vi "Ophir_USBI_Test-2.00.vi"(2 "stop":bool) -> (14 "Power1 (W)":dbl format="%.3p")   [LabVIEW 2012]
panel:
  out "OphirPM":T1
  in  "Wait (mS)":u32=1000
  out "Power2 (W)":dbl(graph)=-5.33e-06
  out "error out":errorcluster
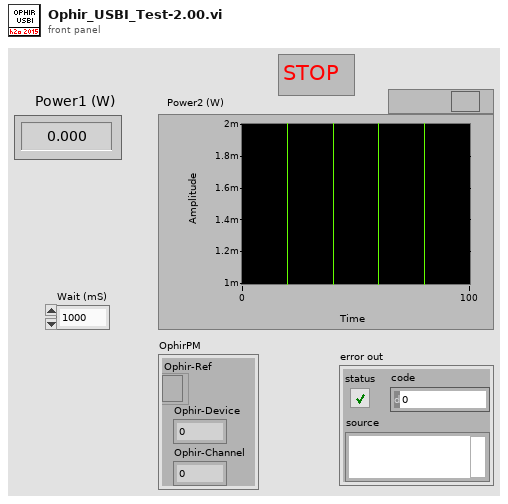
[diagram p1: front panel]
types:
  T1 = cluster{"Ophir-Ref":refnum<k7>, "Ophir-Device":i32, "Ophir-Channel":i32}
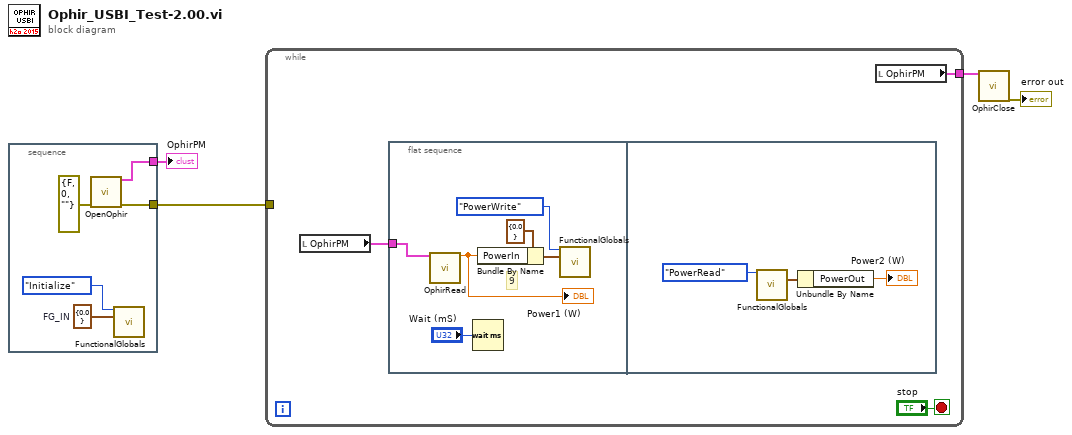
[diagram p0: block diagram]
diagram:
  n1 = stacked-sequence {
    tunnel: [w6] -> w1
    tunnel: [w5] -> w2
    frame #0 {
      w8 = cluster{"PowerIn":dbl} {"PowerIn"=0.0}  # FG_IN
      n2 = call "OpenOphir.vi"("error in (no error)"=errorcluster {"status"=FALSE, "code"=0, "source"=""}) -> ("OphirPM"=w6:T1, "error out"=w5:errorcluster)  [unwired: 13 in]
      n3 = call "FunctionalGlobals.vi"("FG_Control"=enum16{"Initialize", "PowerRead", "PowerWrite"}."Initialize", "FG_IN"=w8) -> ()  [unwired: 13 in, 1 out]
    }
  }
  "OphirPM" <- w1
  n4 = while {
    tunnel: [w12] -> w4
    tunnel: w2 -> [_]
    stop <- "stop" stop-if-true
    n5 = local read "OphirPM"() -> (w10:T1)
    n6 = flat-sequence {
      tunnel: w10 -> [w14]
      frame #0 {
        # "9"
        n7 = call "OphirRead.vi"("OphirPM"=w14) -> ("Power (W)"=w13:dbl)  [unwired: 12 in, 2 out]
        "Power1 (W)" <- w13
        n8 = Wait (ms)(milliseconds to wait="Wait (mS)") -> ()  [unwired: 1 out]
        n9 = Bundle By Name(cluster=cluster{"PowerIn":dbl} {"PowerIn"=0.0} ("FG_IN"), "PowerIn"=w13) -> (w16:cluster{"PowerIn":dbl})
        n10 = call "FunctionalGlobals.vi"("FG_Control"=enum16{"Initialize", "PowerRead", "PowerWrite"}."PowerWrite", "FG_IN"=w16) -> ()  [unwired: 13 in, 1 out]
      }
      frame #1 {
        n11 = call "FunctionalGlobals.vi"("FG_Control"=enum16{"Initialize", "PowerRead", "PowerWrite"}."PowerRead") -> ("FG_OUT"=w20:cluster{"PowerOut":dbl})  [unwired: 14 in]
        n12 = Unbundle By Name(w20) -> ("PowerOut"=→"Power2 (W)":dbl)
      }
    }
    n13 = local read "OphirPM"() -> (w12:T1)
  }
  n14 = call "OphirClose.vi"("OphirPM"=w4) -> ("error out"=→"error out":errorcluster)  [unwired: 18 in]
